vi "fgv_Triggers Output Setup.vi"(6 "Which file? (User profile.ini)":T1=enum."Loaded User profile.ini", 8 "error in (no error)":errorcluster, 10 "Function":T4, 11 "Triggers output setup":T2 {"Pulse width (us)" min=10 max=5000 step=1 format="%.0fµs"}) -> (0 "error out":errorcluster, 3 "Triggers output setup":T2 {"Pulse width (us)" min=10 max=5000 step=1 format="%.0fµs"})   [LabVIEW 2013]
uses:
  Typedefs/HW config states enum.ctl
  Peripherals Control/Triggers/Typedefs/Triggers output setup.ctl
  Peripherals Control/Triggers/Typedefs/Trigger setup element cluster.ctl
  Typedefs/Which path.ctl
  Typedefs/Save-Load enum.ctl
  General Globals.vi
panel:
  # "FUNCTIONAL GLOBAL"
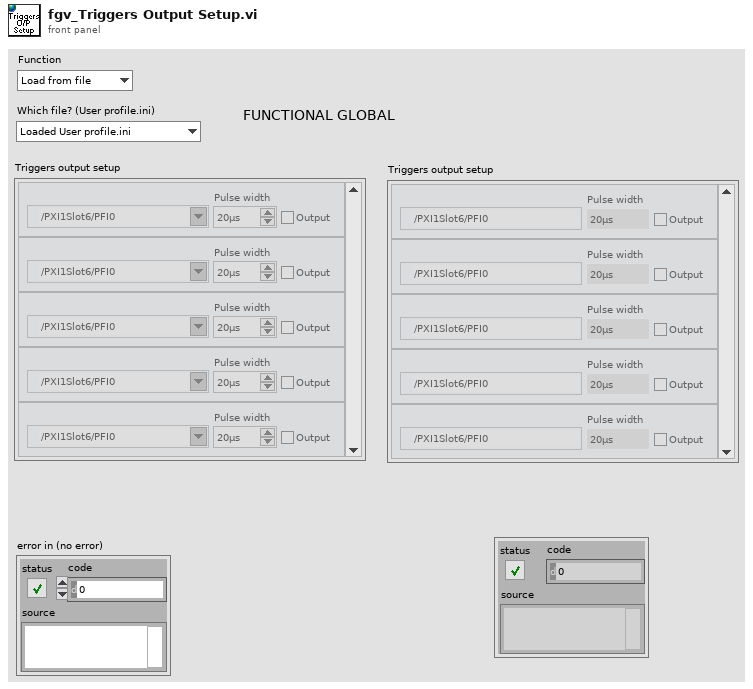
[diagram p1: front panel]
types:
  T1 = typedef "Which path.ctl" = enum16{"Configuration Files", "Calibration Files", "Images", "Setup.ini", "Loaded User profile.ini", "User's-Previous session.ini", "New user profile.ini", "Selected User profile.ini", "User profiles folder", "Power meter scaling.txt", "FOV Cal.ini"}
  T2 = typedef "Triggers output setup.ctl" = T3[]
  T3 = typedef "Trigger setup element cluster.ctl" = cluster{"Name":string, "Output?":bool, "Output terminal":tag, "PXI backplane line":tag, "Pulse width (us)":u16}
  T4 = typedef "HW config states enum.ctl" = enum16{"Load from file", "Save to file", "Write all", "Read all", "Write XY stage settings", "Write DAQ FPGA settings", "Write Control FPGA settings", "Write Phys Channels", "Clear", "Compare from file"}
  T5 = typedef "Save-Load enum.ctl" = enum16{"Save to file", "Load from file", "Compare from file"}
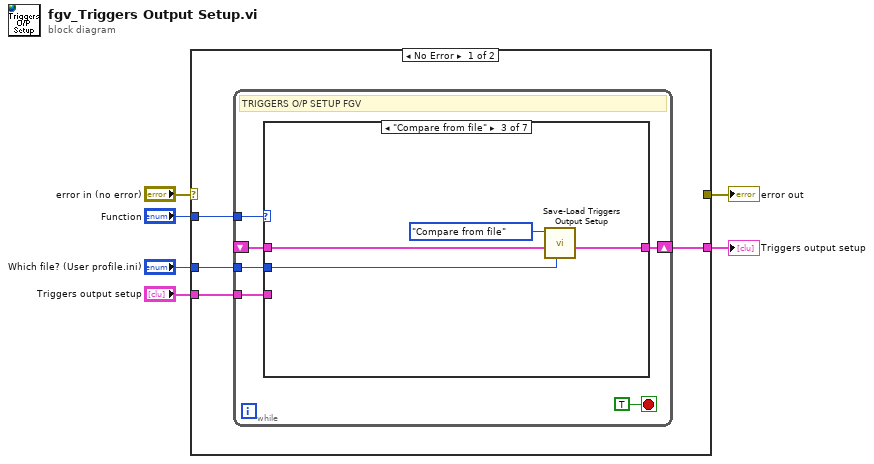
[diagram p0: block diagram]
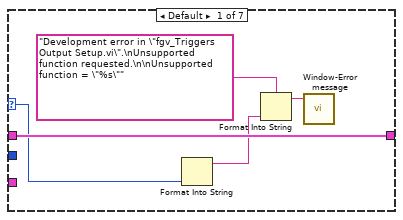
[diagram p2: hidden frame]
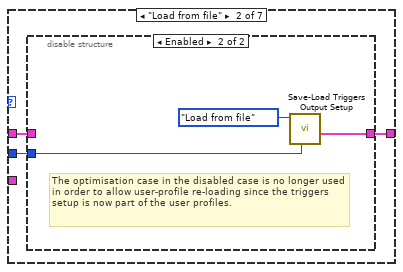
[diagram p3: hidden frame]
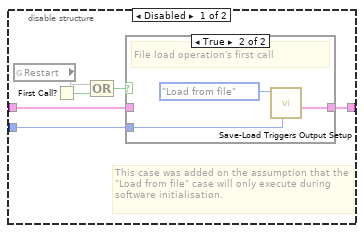
[diagram p4: hidden frame]
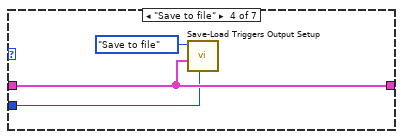
[diagram p6: hidden frame]
diagram:
  n1 = case shown="No Error" "error in (no error)" {
    selector: "error in (no error)" -> [_ w47]
    tunnel: [_ w47] -> w5
    tunnel: "Function" -> [w10 _]
    tunnel: "Triggers output setup" -> [w9 _]
    tunnel: [w8 _] -> w2
    tunnel: "Which file? (User profile.ini)" -> [w7 _]
    frame No Error {
      n2 = while {
        tunnel: w10 -> [w16]
        shift-right: [w14] -> w8
        shift-left: _ -> [w12]
        tunnel: w9 -> [w13]
        tunnel: w7 -> [w11]
        stop <- TRUE stop-if-true
        # "TRIGGERS O/P SETUP FGV"
        n3 = case shown="\"Compare from file\"" w16 {
          selector: w16 -> [w20 _ _ _ _ _ _]
          tunnel: [w21 w24 w41 w43 w45 w46 _] -> w14
          tunnel: w13 -> [_ _ _ _ w45 _ _]
          tunnel: w12 -> [w21 w23 w38 w43 _ w46 _]
          tunnel: w11 -> [_ w22 w40 w42 _ _ _]
          frame Default {
            n4 = Format Into String(w20) -> (resulting string=w18:string)  [unwired: 3 in, 1 out]
            n5 = Format Into String(format string="Development error in \"fgv_Triggers Output Setup.vi\".\nUnsupported function requested.\n\nUnsupported function = \"%s\"" ("Message"), w18) -> (resulting string=w17:string)  [unwired: 2 in, 1 out]
            n6 = call "Window-Error message.vi"("Message"=w17) -> ()  [unwired: 10 in, 1 out]
          }
          frame "Load from file" {
            n7 = disable-structure shown="Enabled" {
              disable-tunnel: [w30 w37] -> w24
              disable-tunnel: w23 -> [w29 _]
              disable-tunnel: w22 -> [w25 w36]
              frame Disabled {
                # "This case was added on the assumption that the \"Load from file\" case will only execute during software initialisation."
                n8 = global read "General Globals.vi" "Restart"() -> (w27)
                n9 = First Call?() -> (First Call?: T/F=w28:bool)
                n10 = Compound Arithmetic op=OR(w27, w28) -> (w26:bool)
                n11 = case shown="True" w26 {
                  tunnel: [w31 w34] -> w30
                  tunnel: w29 -> [w31 _]
                  tunnel: w25 -> [_ w32]
                  frame False {
                    # "Already loaded"
                  }
                  frame True {
                    # "File load operation's first call"
                    n12 = call "Save-Load Triggers Output Setup.vi"("Which file? (User profile.ini)"=w32, "Function"=Save-Load_enum."Load from file") -> ("Triggers output setup"=w34:T2)  [unwired: 8 in, 1 out]
                  }
                }
              }
              frame Enabled {
                # "The optimisation case in the disabled case is no longer used in order to allow user-profile re-loading since the triggers setup is now part of the user profiles."
                n13 = call "Save-Load Triggers Output Setup.vi"("Which file? (User profile.ini)"=w36, "Function"=Save-Load_enum."Load from file") -> ("Triggers output setup"=w37:T2)  [unwired: 8 in, 1 out]
              }
            }
          }
          frame "Compare from file" {
            n14 = call "Save-Load Triggers Output Setup.vi"("Which file? (User profile.ini)"=w40, "Triggers output setup to save"=w38, "Function"=Save-Load_enum."Compare from file") -> ("Triggers output setup"=w41:T2)  [unwired: 7 in, 1 out]
          }
          frame "Save to file" {
            n15 = call "Save-Load Triggers Output Setup.vi"("Which file? (User profile.ini)"=w42, "Triggers output setup to save"=w43, "Function"=Save-Load_enum."Save to file") -> ()  [unwired: 7 in, 2 out]
          }
          frame "Write all" {
          }
          frame "Read all" {
          }
          frame "Clear" {
          }
        }
      }
    }
    frame Error {
    }
  }
  "error out" <- w5
  "Triggers output setup" <- w2
